vi "PH_DeformableMirror.destructor.vi"(0 "i ref in":refnum<vi>, 5 "error in(no error)":errorcluster) -> (19 "error out":errorcluster)   [LabVIEW 2014, in "PH_DeformableMirror.lvlib"]
doc: "This is the destructor of a class.\n\nLicense Agreement for this software:\n\nCopyright (C)\nGesellschaft für Schwerionenforschung, GSI\nPlanckstr. 1\n64291 Darmstadt\nGermany\n\nContact: D.Beck@gsi.de \n\nThis program is free software; you can redistribute it and/or modify it under the terms of the \nGNU General Public License as published by the Free Software Foundation; either version 2 of \nthe license, or (at your option) any later version.\n\nThis program is distributed in the hope that it will be useful, but WITHOUT ANY WARRANTY; \nwithout even the implied warranty of MERCHANTABILITY or FITNESS FOR A PARTICULAR PURPOSE. See the GNU General License for more details (http://www.gnu.org).\n\nGesellschaft für Schwerionenforschung, GSI\nPlanckstr. 1, 64291 Darmstadt, Germany\nFor all questions and ideas contact: M.Richter@gsi.de, H.Brand@gsi.de or D.Beck@gsi.de.\nLast update: 16-JUN-2004"
uses:
  PH_DeformableMirror.lvlib
  PH_StatusHandler/PH_StatusHandler.lvlib
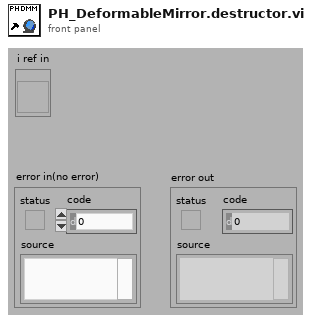
[diagram p1: front panel]
types:
  T1 = enum16{"SetAttribute", "GetAttribute", "CreateAttribute", "DestroyAttribute", "DestroyAllAtributes"}
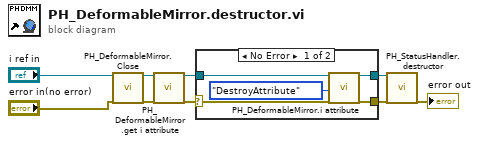
[diagram p0: block diagram]
diagram:
  n1 = call "PH_DeformableMirror.Close.vi"("VI in"="i ref in", "error in (no error)"="error in(no error)") -> ("VI out"=w3:refnum<vi>, "error out"=w5:errorcluster)  [unwired: 16 in]
  n2 = call "PH_DeformableMirror.get i attribute.vi"("i ref in"=w3, "error in (no error)"=w5) -> ("i ref out"=w9:refnum<vi>, "error out"=w1:errorcluster)  [unwired: 15 in, 1 out]
  n3 = case shown="No Error" w1 {
    selector: w1 -> [w10 w15]
    tunnel: w9 -> [w14 w16]
    tunnel: [w12 w15] -> w8
    tunnel: [w11 w16] -> w6
    frame No Error {
      n4 = call "PH_DeformableMirror.i attribute.vi"("VI Refnum"=w14, "Action"=T1."DestroyAttribute", "error in (no error)"=w10) -> ("VI Refnum out"=w11:refnum<vi>, "error out"=w12:errorcluster)  [unwired: 14 in, 1 out]
    }
    frame Error {
    }
  }
  n5 = call "PH_StatusHandler.destructor.vi"("i ref in"=w6, "error in(no error)"=w8) -> ("error out"=→"error out":errorcluster)  [unwired: 17 in]
